vi "AutoUpdate.vi"() -> ()   [LabVIEW 2025]
uses:
  D:/LV test/LabVIEWConfigSecurity.dll
  LabVIEWConfigSecurity.dll
panel:
  out "UpdateInspectionTime":bool
  in  "stationName":string
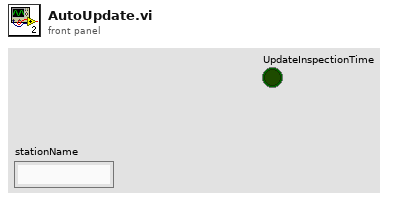
[diagram p1: front panel]
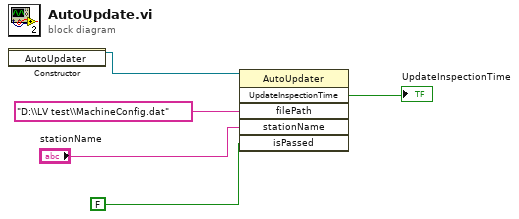
[diagram p0: block diagram]
diagram:
  n1 = constructor class="AutoUpdater"() -> (reference out=w5:refnum<k24>)  [unwired: 3 in, 2 out]
  n2 = invoke on="调用节点" class="AutoUpdater" method="UpdateInspectionTime"(reference=w5, "filePath"="D:\\LV test\\MachineConfig.dat", "stationName"="stationName", "isPassed"=FALSE) -> ("UpdateInspectionTime"=→"UpdateInspectionTime":bool)  [unwired: 2 in, 5 out]
